vi "Telescope Test Program.vi"() -> ()   [LabVIEW 2019]
uses:
  Telescope cluster Status.ctl
  typedefs/CC cluster RA and DEC.ctl
  Telescope enum Status.ctl
  Telescope cluster Settings.ctl
  Telescope.lvclass
  <vilib>/Utility/sysdir.llb/System Directory Type.ctl
  PRIME Telescope/PRIME Telescope cluster Settings.ctl
panel:
  out "Log File":path
  in  "Polling Rate (seconds)":dbl=5.0
  out "Raw Response From Telescope":string
  in  "Telescope Type":u16(ring) items=["PRIME", "Simulator"]
  in  "Connect":bool
  out "error":errorcluster
  out "Connected":bool
  in  "remote port":u16=8766
  in  "IP Address":string="192.168.12.98"
  in  "Telescope Settings":T1
  in  "Begin Move":bool
  in  "Position":T2
  out "Telescope Status":T3
  in  "Close":bool
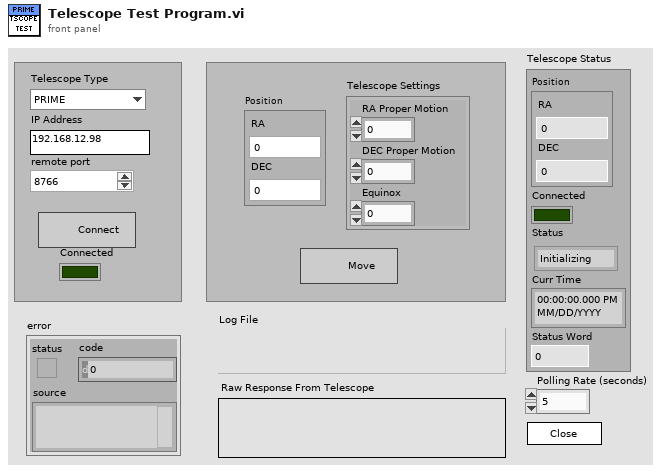
[diagram p1: front panel]
types:
  T1 = typedef "Telescope cluster Settings.ctl" = cluster{"RA Proper Motion":dbl, "DEC Proper Motion":dbl, "Equinox":dbl}
  T2 = typedef "CC cluster RA and DEC.ctl" = cluster{"RA":dbl, "DEC":dbl}
  T3 = typedef "Telescope.lvclass/Telescope cluster Status.ctl" = cluster{"Position":T2, "Connected":bool, "Status":T4, "Curr Time":timestamp, "Status Word":u32}
  T4 = typedef "Telescope.lvclass/Telescope enum Status.ctl" = enum16{"Initializing", "Ready", "Moving", "Error"}
  T5 = cluster{"state":refnum<user-event>, "Telescope Name":string, "Telescope ref":refnum<class "Telescope.lvclass">, "init parameters":variant, "poll":bool, "log file":refnum<file>}
  T6 = enum16{"open", "replace", "create", "open or create", "replace or create", "replace or create with confirmation"}
  T7 = typedef "PRIME Telescope cluster Settings.ctl" = cluster{"IP Address":string, "port":u16}
  T8 = typedef "System Directory Type.ctl" = i32
  T9 = typedef "CC cluster Hardware Config.ctl" = cluster{"Filter Wheel Name":string, "Defined Filter Wheels":string[], "Telescope Name":string, "Defined Telescopes":string[], "CryoServer Name":string, "Defined CryoServers":string[]}
  T10 = enum32{"invalid app kind", "Development System", "Run Time System", "Student Edition", "Embedded LabVIEW", "Evaluation", "Custom"}
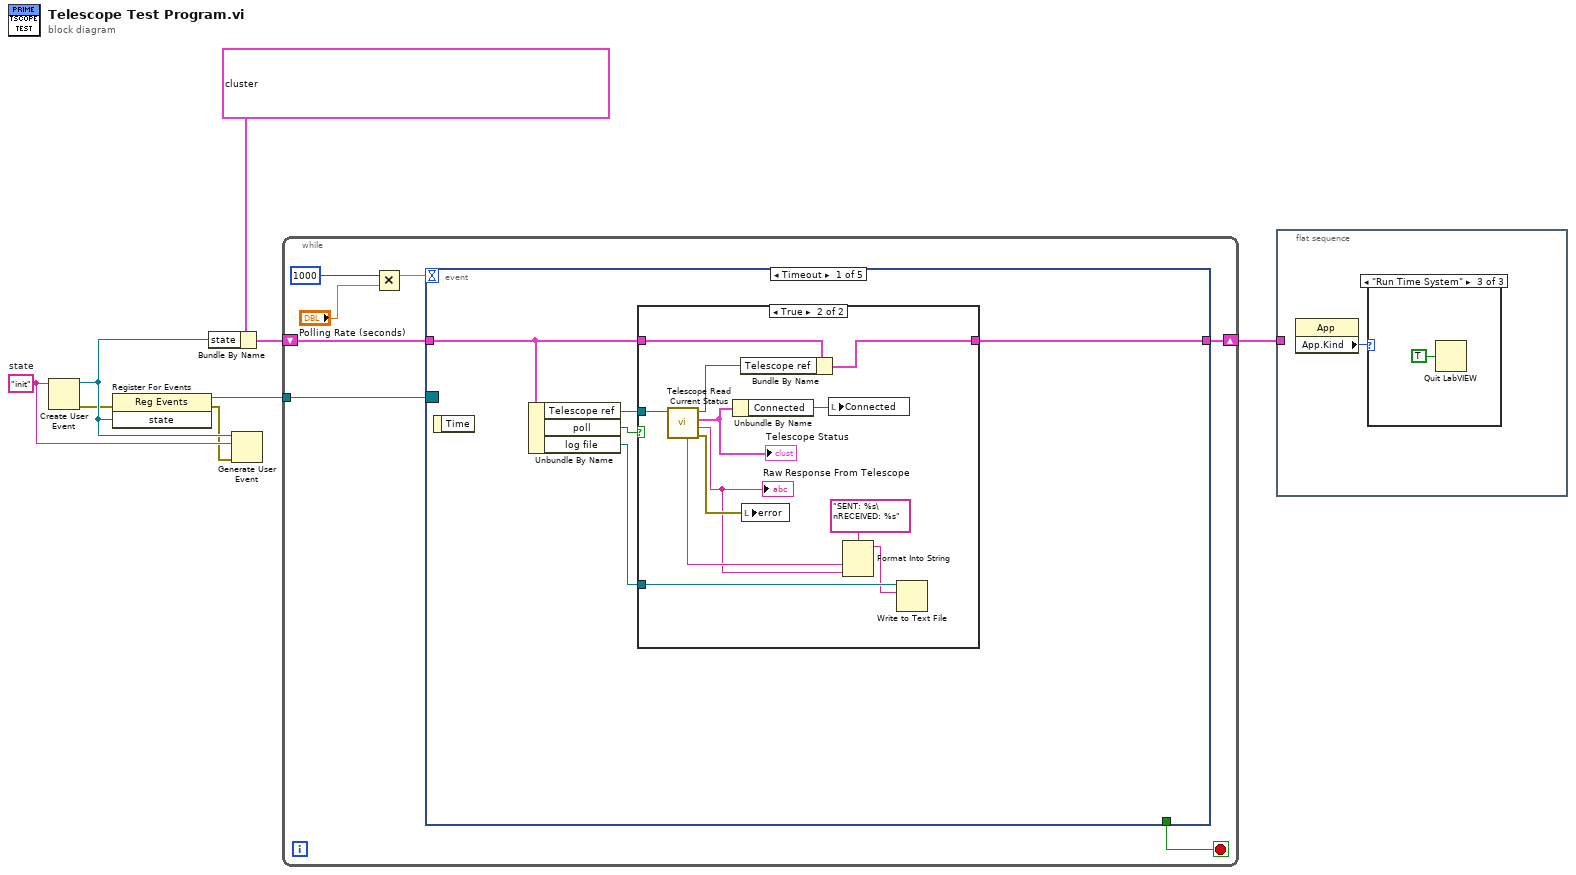
[diagram p0: block diagram]
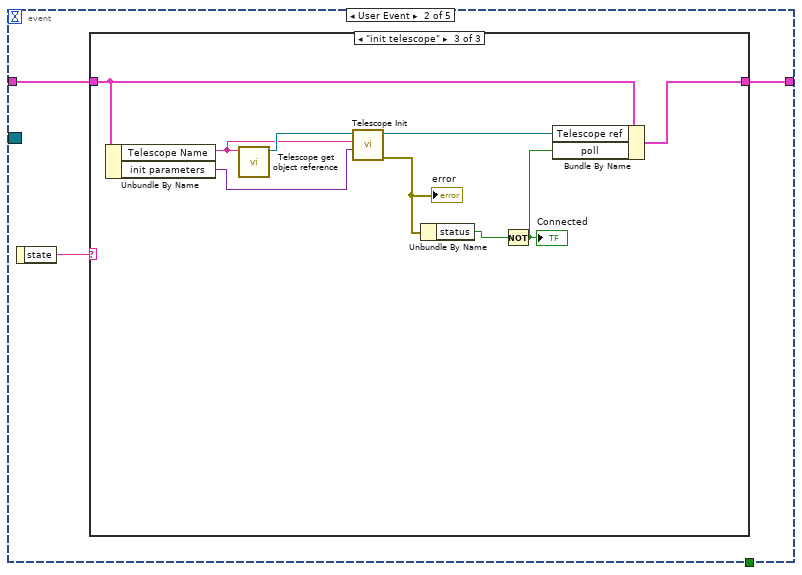
[diagram p5: hidden frame]
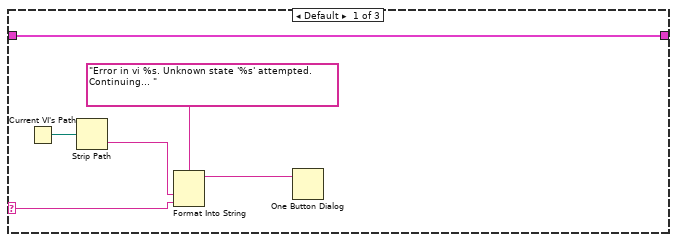
[diagram p6: hidden frame]
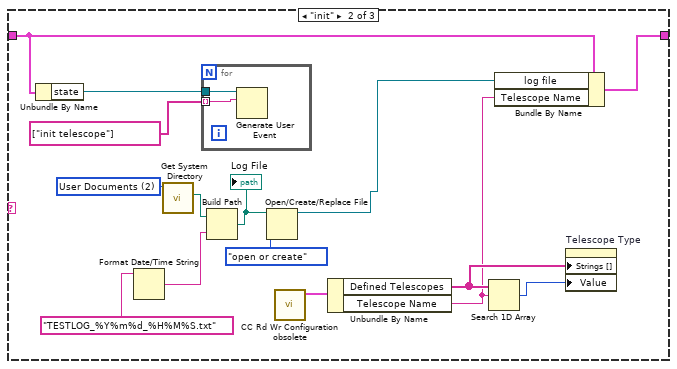
[diagram p7: hidden frame]
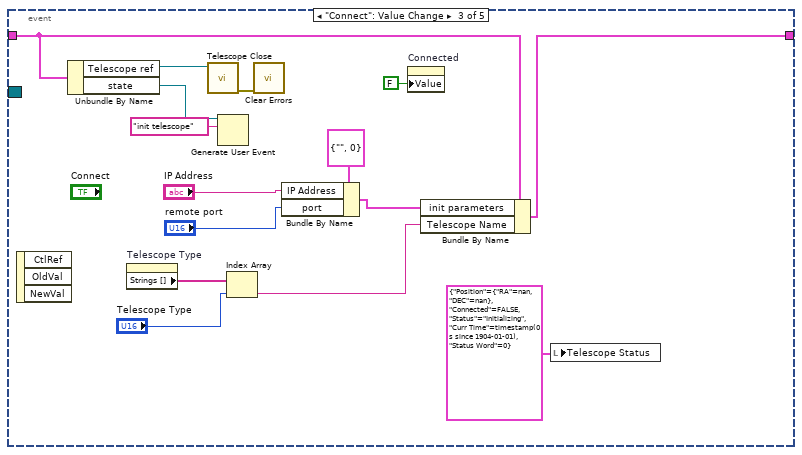
[diagram p8: hidden frame]
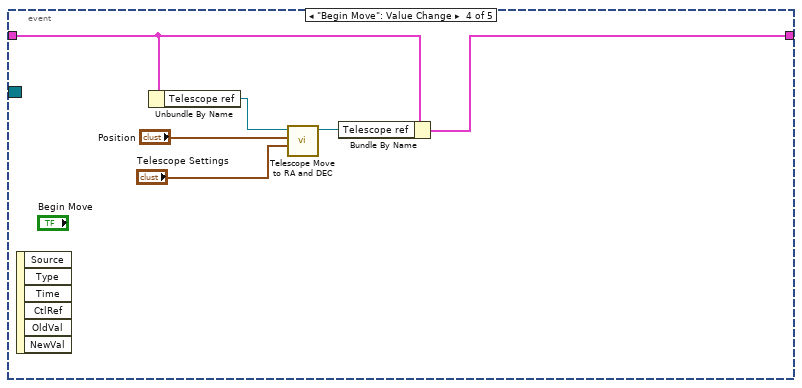
[diagram p9: hidden frame]
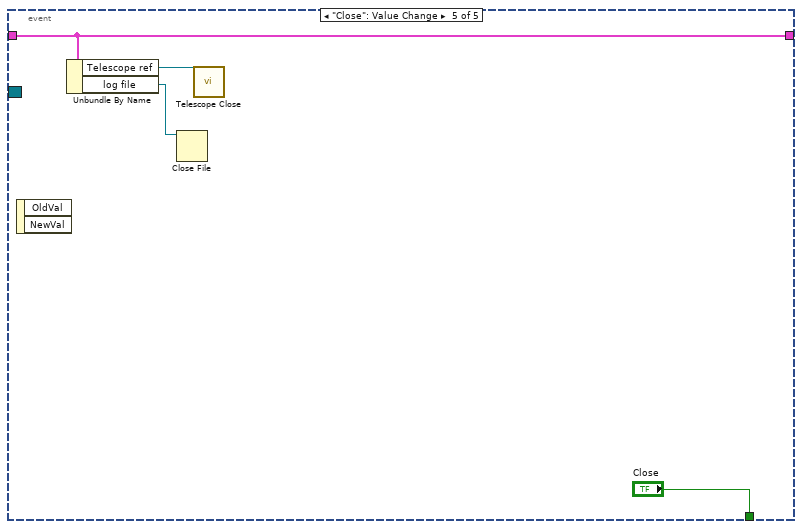
[diagram p10: hidden frame]
diagram:
  w4 = "init"  # state
  n1 = Create User Event(user event datatype=w4) -> (user event=w6:refnum<user-event>, error out=w2:errorcluster)  [unwired: 1 in]
  n2 = register-events(error in=w2, w6) -> (reference out=w5:refnum<event-registration>, error out=w3:errorcluster)  [unwired: 1 in]
  n3 = Bundle By Name(cluster=T5 {"state"=refnum, "Telescope Name"="", "Telescope ref"=refnum, "init parameters"=variant, "poll"=FALSE, "log file"=refnum}, "state"=w6) -> (w7:T5)
  n4 = Generate User Event(user event=w6, event data cluster=w4, error in=w3) -> ()  [unwired: 1 in, 2 out]
  n5 = while {
    tunnel: w5 -> [w15]
    shift-right: [w13] -> w1
    shift-left: w7 -> [w14]
    stop <- w12 stop-if-true
    n6 = Multiply(x=1000, y="Polling Rate (seconds)") -> (x*y=w10:dbl)
    n7 = event shown="[0] Timeout" {
      selector: w15 -> [_ _ _ _ _]
      dyn-events: _ -> [_ _ _ _ _]
      timeout: w10 -> [_ _ _ _ _]
      tunnel: w14 -> [w18 w35 w80 w84 w92]
      tunnel: [w17 w34 w81 w85 w92] -> w13
      tunnel: [_ _ _ _ "Close"] -> w12
      event Timeout {
        n8 = event-data() -> ()  [unwired: 1 in, 1 out]
        n9 = Unbundle By Name(w18) -> ("Telescope ref"=w20:refnum<class "Telescope.lvclass">, "poll"=w19:bool, "log file"=w16:refnum<file>)
        n10 = case shown="True" w19 {
          tunnel: w20 -> [_ w33]
          tunnel: w18 -> [w21 w32]
          tunnel: [w21 w30] -> w17
          tunnel: w16 -> [_ w28]
          frame False {
          }
          frame True {
            n11 = call-dynamic "Telescope Read Current Status.vi"("Telescope in"=w33) -> ("error out"=w29:errorcluster, "Raw Response"=w25:string, "Telescope Status"=w23:T3, "Telescope out"=w31:refnum<class "Telescope.lvclass">, "Cmd Sent"=w26:string)  [unwired: 6 in]
            "Telescope Status" <- w23
            "Raw Response From Telescope" <- w25
            n12 = Unbundle By Name(w23) -> ("Connected"=w22:bool)
            n13 = Bundle By Name(cluster=w32, "Telescope ref"=w31) -> (w30:T5)
            n14 = local write "error"(w29) -> ()
            n15 = local write "Connected"(w22) -> ()
            n16 = Format Into String(format string="SENT: %s\nRECEIVED: %s", w26, w25) -> (resulting string=w24:string)  [unwired: 2 in, 1 out]
            n17 = Write to Text File(file (use dialog)=w28, text=w24) -> ()  [unwired: 2 in, 3 out]
          }
        }
      }
      event User Event {
        n18 = event-data() -> ("state"=w36:string)  [unwired: 1 in]
        n19 = case shown="\"init telescope\"" w36 {
          selector: w36 -> [w41 _ _]
          tunnel: w35 -> [w37 w50 w67]
          tunnel: [w37 w51 w68] -> w34
          frame Default {
            n20 = Current VI's Path() -> (path=w40:path)
            n21 = Strip Path(path=w40) -> (name=w39:string)  [unwired: 1 out]
            n22 = Format Into String(format string="Error in vi %s. Unknown state '%s' attempted. Continuing... ", w39, w41) -> (resulting string=w38:string)  [unwired: 2 in, 1 out]
            n23 = One Button Dialog(message=w38) -> ()  [unwired: 1 in, 1 out]
          }
          frame "init" {
            w48 = T8 2 items=["User Home"=0, "User Desktop"=1, "User Documents"=2, "User Application Data"=3, "User Preferences"=4, "User Temporary"=5, "Public Documents"=6, "Public Application Data"=7, "Public Preferences"=8, "Public Cache"=13, "System Core Libraries"=9, "System Installed Libraries"=10, "Application Files"=11, "Boot Volume Root"=12] ("system directory type")
            n24 = Unbundle By Name(w50) -> ("state"=w54:refnum<user-event>)
            n25 = Format Date/Time String(time format string (%c)="TESTLOG_%Y%m%d_%H%M%S.txt") -> (date/time string=w46:string)  [unwired: 2 in]
            n26 = call <vilib>:"Get System Directory.vi"("system directory type"=w48) -> ("system directory"=w47:path)  [unwired: 10 in]
            n27 = for {
              tunnel: w54 -> [w59]
              tunnel: string[] ["init telescope"] -> [w58] mode=indexing
              n28 = Generate User Event(user event=w59, event data cluster=w58) -> ()  [unwired: 2 in, 2 out]
            }
            n29 = Build Path(base path=w47, name or relative path=w46) -> (appended path=w45:path)
            "Log File" <- w45
            n30 = Open/Create/Replace File(file path (use dialog)=w45, operation (0:open)=T6."open or create") -> (refnum out=w43:refnum<file>)  [unwired: 4 in, 2 out]
            n31 = call "CC Rd Wr Configuration obsolete.vi"() -> ("Hardware Config out"=w57:T9)  [unwired: 10 in, 1 out]
            n32 = Unbundle By Name(w57) -> ("Defined Telescopes"=w55:string[], "Telescope Name"=w52:string)
            n33 = Search 1D Array(1D array=w55, element=w52) -> (index of element=w56:i32)  [unwired: 1 in]
            n34 = Bundle By Name(cluster=w50, "log file"=w43, "Telescope Name"=w52) -> (w51:T5)
            n35 = property on="Telescope Type" class="Ring (strict)"("Strings []"=w55, "Value"=w56) -> ()  [unwired: 2 in, 2 out]
          }
          frame "init telescope" {
            n36 = Unbundle By Name(w67) -> ("Telescope Name"=w63:string, "init parameters"=w61:variant)
            n37 = call "Telescope get object reference.vi"("Telescope Name"=w63) -> ("PRIME Telescope.lvclass"=w65:refnum<class "Telescope.lvclass">)  [unwired: 8 in, 2 out]
            n38 = call-dynamic "Telescope Init.vi"("Settings"=w61, "Name"=w63, "Telescope in"=w65) -> ("error out"=w62:errorcluster, "Telescope out"=w64:refnum<class "Telescope.lvclass">)  [unwired: 6 in, 1 out]
            "error" <- w62
            n39 = Unbundle By Name(w62) -> ("status"=w66:bool)
            n40 = Not(x=w66) -> (.not. x?=w60:bool)
            "Connected" <- w60
            n41 = Bundle By Name(cluster=w67, "Telescope ref"=w64, "poll"=w60) -> (w68:T5)
          }
        }
      }
      event "Connect": Value Change {
        n42 = event-data() -> ()  [unwired: 1 in, 3 out]
        n43 = Unbundle By Name(w80) -> ("Telescope ref"=w79:refnum<class "Telescope.lvclass">, "state"=w78:refnum<user-event>)
        n44 = property on="Telescope Type" class="Ring (strict)"() -> ("Strings []"=w83:string[])  [unwired: 2 in, 2 out]
        n45 = call-dynamic "Telescope Close.vi"("Telescope in"=w79) -> ("error out"=w71:errorcluster)  [unwired: 9 in, 1 out]
        n46 = Generate User Event(user event=w78, event data cluster="init telescope" ("event data")) -> ()  [unwired: 2 in, 2 out]
        n47 = Index Array(array=w83, index="Telescope Type") -> (element=w82:string)
        n48 = call <vilib>:"Clear Errors.vi"("error in (no error)"=w71) -> ()  [unwired: 5 in, 2 out]
        n49 = Bundle By Name(cluster=T7 {"IP Address"="", "port"=0} ("Settings"), "IP Address"="IP Address", "port"="remote port") -> (w72:T7)
        n50 = property on="Connected" class="Bool (strict)"("Value"=FALSE ("Connected")) -> ()  [unwired: 2 in, 2 out]
        n51 = Bundle By Name(cluster=w80, "init parameters"=w72, "Telescope Name"=w82) -> (w81:T5)
        n52 = local write "Telescope Status"(T3 {"Position"={"RA"=nan, "DEC"=nan}, "Connected"=FALSE, "Status"=enum."Initializing", "Curr Time"=timestamp(0 s since 1904-01-01), "Status Word"=0} ("Telescope Status")) -> ()
      }
      event "Begin Move": Value Change {
        n53 = event-data() -> ()  [unwired: 1 in, 6 out]
        n54 = Unbundle By Name(w84) -> ("Telescope ref"=w89:refnum<class "Telescope.lvclass">)
        n55 = call-dynamic "Telescope Move to RA and DEC.vi"("Target Info"="Telescope Settings", "RA and DEC"="Position", "Telescope in"=w89) -> ("Telescope out"=w86:refnum<class "Telescope.lvclass">)  [unwired: 7 in, 1 out]
        n56 = Bundle By Name(cluster=w84, "Telescope ref"=w86) -> (w85:T5)
      }
      event "Close": Value Change {
        n57 = event-data() -> ()  [unwired: 1 in, 2 out]
        n58 = Unbundle By Name(w92) -> ("Telescope ref"=w91:refnum<class "Telescope.lvclass">, "log file"=w90:refnum<file>)
        n59 = Close File(refnum=w90) -> ()  [unwired: 1 in, 2 out]
        n60 = call-dynamic "Telescope Close.vi"("Telescope in"=w91) -> ()  [unwired: 9 in, 2 out]
      }
    }
  }
  n61 = flat-sequence {
    tunnel: w1 -> [_]
    frame #0 {
      n62 = property class="App"() -> ("App.Kind"=w94:T10)  [unwired: 2 in, 2 out]
      n63 = case shown="\"Run Time System\"" w94 {
        frame "invalid app kind", Default {
        }
        frame "Development System" {
        }
        frame "Run Time System" {
          n64 = Quit LabVIEW(quit? (T)=TRUE) -> ()
        }
      }
    }
  }
